vi "DSF.Engine.Pool.Get FIFO.vi"(11 "Pool in":refnum<class "DSF.Engine.Pool.lvclass">) -> (2 "FIFO":refnum<k33>, 3 "Pool out":refnum<class "DSF.Engine.Pool.lvclass">)   [LabVIEW 2017, in "DSF.Engine.lvlib" / "DSF.Engine.Pool.lvclass"]
uses:
  DSF.Engine.Pool.lvclass
  DSF.Engine.Pool.lvclass/DSF.Engine.Pool.ctl
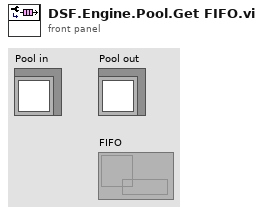
[diagram p1: front panel]
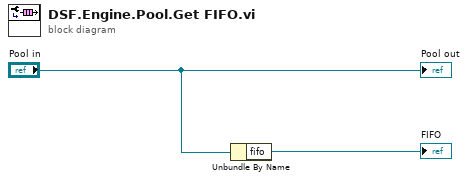
[diagram p0: block diagram]
diagram:
  n1 = Unbundle By Name("Pool in") -> ("fifo"=→"FIFO":refnum<k33>)
  "Pool out" <- "Pool in"
